vi "getClientID.vi"(11 "CONNECT in":refnum<class "CONNECT.lvclass">) -> (2 "Client ID":string, 3 "CONNECT out":refnum<class "CONNECT.lvclass">)   [LabVIEW 2013, in "MQTT_Control_Packets.lvlib" / "CONNECT.lvclass"]
uses:
  CONNECT.lvclass
  ControlPacket/ControlPacket.lvclass/ControlPacket.ctl
  ControlPacket/ControlPacket.lvclass
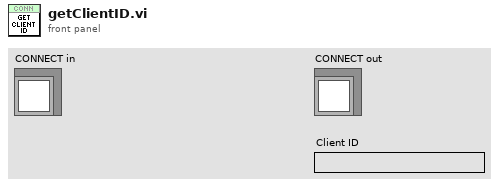
[diagram p1: front panel]
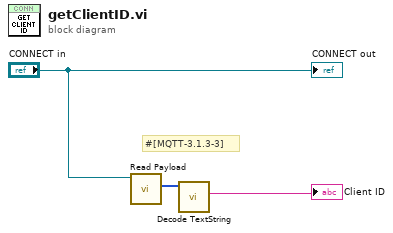
[diagram p0: block diagram]
diagram:
  # "#[MQTT-3.1.3-3]"
  n1 = call "Read Payload.vi"("ControlPacket in"="CONNECT in") -> ("Payload"=w3:u8[])  [unwired: 9 in, 1 out]
  n2 = call "Decode TextString.vi"("Length-Prefixed Field"=w3) -> ("Text String"=→"Client ID":string)  [unwired: 8 in, 2 out]
  "CONNECT out" <- "CONNECT in"
